vi "JSON type.vi"(10 "Offset":i32, 11 "JSON":string) -> (2 "Item Offset":i32, 3 "JSON Value Type":T1)   [LabVIEW 2024, in "JSONtext.lvlib"]
doc: "Determines the type of a JSON Value (object, array, string, number, true, false, or null)\n\n\"Offset\" should point to the start of the JSON Value, or to whitespace in front of the Value.\n\nThis function does not do a full validation of the Value, but instead identifies it only from its start (so, for example, something starting with \"{\" will be identified as a JSON Object)."
uses:
  JSONtext.lvlib
  JSON Value Type.ctl
  Advance past whitespace.vi
  Advance past Number.vi
  Advance past Line Ending.vi
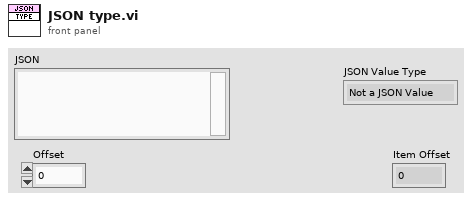
[diagram p1: front panel]
types:
  T1 = typedef "JSONtext.lvlib/JSON Value Type.ctl" = enum16{"Not a JSON Value", "JSON Object", "JSON Array", "String", "Number", "true", "false", "null"}
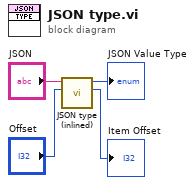
[diagram p0: block diagram]
diagram:
  n1 = call "JSON type (inlined).vi"("Offset"="Offset", "JSON"="JSON") -> ("Item Offset"=→"Item Offset":i32, "JSON Value Type"=→"JSON Value Type":T1)  [unwired: 8 in]
